vi "Axis Column.vi"() -> ()   [LabVIEW 2026]
panel:
  in  "stop":bool
  out "appended path":path
  out "name":string
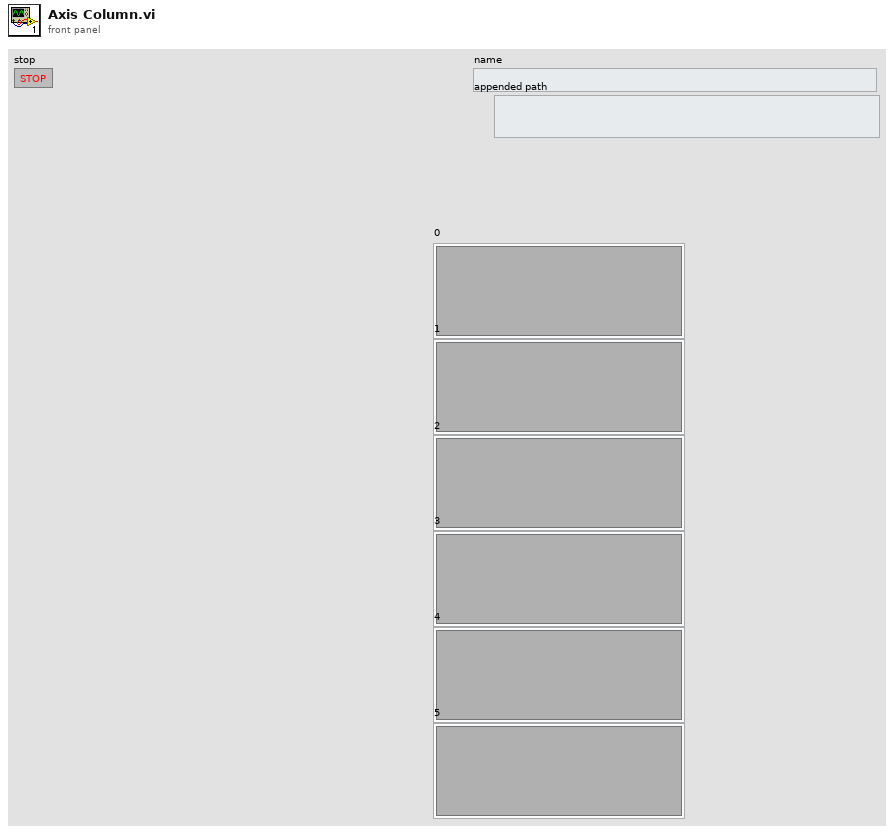
[diagram p1: front panel]
types:
  T1 = cluster{"[0]":refnum<vi>, "[1]":refnum<vi>, "[2]":refnum<vi>, "[3]":refnum<vi>, "[4]":refnum<vi>, "[5]":refnum<vi>, "[6]":refnum<vi>, "[7]":refnum<vi>, "[8]":refnum<vi>}
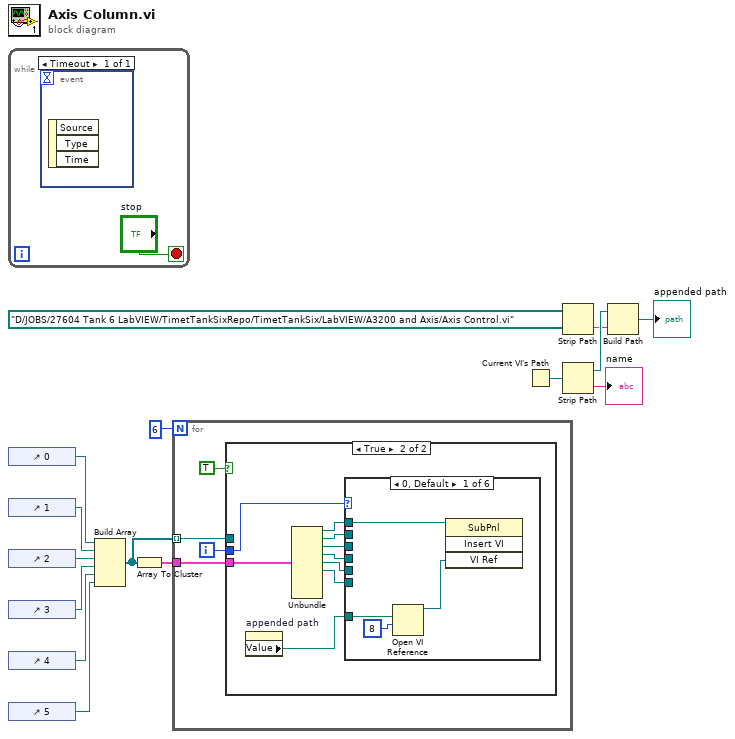
[diagram p0: block diagram]
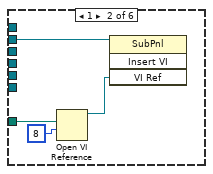
[diagram p3: hidden frame]
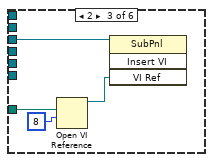
[diagram p4: hidden frame]
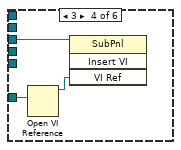
[diagram p5: hidden frame]
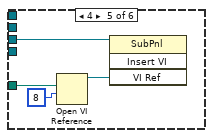
[diagram p6: hidden frame]
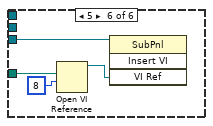
[diagram p7: hidden frame]
diagram:
  n1 = while {
    stop <- "stop" stop-if-true
    n2 = event shown="[0] Timeout" {
      selector: _ -> [_]
      dyn-events: _ -> [_]
      timeout: _ -> [_]
      event Timeout {
        n3 = event-data() -> ()  [unwired: 1 in, 3 out]
      }
    }
  }
  n4 = control-ref of="0"() -> (w8:refnum<vi>)
  n5 = control-ref of="1"() -> (w7:refnum<vi>)
  n6 = control-ref of="2"() -> (w6:refnum<vi>)
  n7 = control-ref of="3"() -> (w5:refnum<vi>)
  n8 = control-ref of="4"() -> (w4:refnum<vi>)
  n9 = control-ref of="5"() -> (w3:refnum<vi>)
  n10 = Build Array(w8, w7, w6, w5, w4, w3) -> (w2:refnum<vi>[])
  n11 = Array To Cluster(array=w2) -> (cluster=w1:T1)
  n12 = for {
    N: 6 -> [_]
    tunnel: w2 -> [w19] mode=indexing
    tunnel: w1 -> [w17]
    i -> [w18]
    n13 = case shown="True" TRUE {
      tunnel: w19 -> [_ _]
      tunnel: w18 -> [_ w29]
      tunnel: w17 -> [_ w27]
      frame False {
      }
      frame True {
        n14 = property on="appended path" class="Path"() -> ("Value"=w28:path)  [unwired: 2 in, 2 out]
        n15 = Unbundle(w27) -> ("[0]"=w26:refnum<vi>, "[1]"=w25:refnum<vi>, "[2]"=w24:refnum<vi>, "[3]"=w23:refnum<vi>, "[4]"=w22:refnum<vi>, "[5]"=w21:refnum<vi>)  [unwired: 3 out]
        n16 = case shown="0, Default" w29 {
          tunnel: w28 -> [w33 w37 w40 w44 w48 w52]
          tunnel: w26 -> [w31 _ _ _ _ _]
          tunnel: w25 -> [_ w35 _ _ _ _]
          tunnel: w24 -> [_ _ w39 _ _ _]
          tunnel: w23 -> [_ _ _ w42 _ _]
          tunnel: w22 -> [_ _ _ _ w46 _]
          tunnel: w21 -> [_ _ _ _ _ w50]
          frame 0, Default {
            n17 = Open VI Reference(vi path=w33, options=8) -> (vi reference=w32:refnum<vi>)  [unwired: 4 in, 1 out]
            n18 = invoke on="Invoke Node" class="SubPnl" method="Insert VI"(reference=w31, "VI Ref"=w32) -> ()  [unwired: 2 in, 4 out]
          }
          frame 1 {
            n19 = Open VI Reference(vi path=w37, options=8) -> (vi reference=w36:refnum<vi>)  [unwired: 4 in, 1 out]
            n20 = invoke on="Invoke Node" class="SubPnl" method="Insert VI"(reference=w35, "VI Ref"=w36) -> ()  [unwired: 2 in, 4 out]
          }
          frame 2 {
            n21 = Open VI Reference(vi path=w40, options=8) -> (vi reference=w41:refnum<vi>)  [unwired: 4 in, 1 out]
            n22 = invoke on="Invoke Node" class="SubPnl" method="Insert VI"(reference=w39, "VI Ref"=w41) -> ()  [unwired: 2 in, 4 out]
          }
          frame 3 {
            n23 = Open VI Reference(vi path=w44) -> (vi reference=w43:refnum<vi>)  [unwired: 5 in, 1 out]
            n24 = invoke on="Invoke Node" class="SubPnl" method="Insert VI"(reference=w42, "VI Ref"=w43) -> ()  [unwired: 2 in, 4 out]
          }
          frame 4 {
            n25 = Open VI Reference(vi path=w48, options=8) -> (vi reference=w47:refnum<vi>)  [unwired: 4 in, 1 out]
            n26 = invoke on="Invoke Node" class="SubPnl" method="Insert VI"(reference=w46, "VI Ref"=w47) -> ()  [unwired: 2 in, 4 out]
          }
          frame 5 {
            n27 = Open VI Reference(vi path=w52, options=8) -> (vi reference=w51:refnum<vi>)  [unwired: 4 in, 1 out]
            n28 = invoke on="Invoke Node" class="SubPnl" method="Insert VI"(reference=w50, "VI Ref"=w51) -> ()  [unwired: 2 in, 4 out]
          }
        }
      }
    }
  }
  n29 = Current VI's Path() -> (path=w15:path)
  n30 = Strip Path(path=path "D:/JOBS/27604 Tank 6 LabVIEW/TimetTankSixRepo/TimetTankSix/LabVIEW/A3200 and Axis/Axis Control.vi") -> (name=w10:string)  [unwired: 1 out]
  n31 = Strip Path(path=w15) -> (stripped path=w13:path, name=→"name":string)
  n32 = Build Path(base path=w13, name or relative path=w10) -> (appended path=→"appended path":path)
